vi "Multiple read.vi"(8 "error in (no error)":errorcluster, 9 "Data In":variant[](array[variant]), 10 "Section Names":string[](array[string]), 11 "Configuration File in":refnum<class "Configuration File.lvclass">) -> (0 "error out":errorcluster, 1 "Found section and keys?":bool[](array[boolean]), 2 "Data Out":variant[](array[variant]), 3 "Configuration File out":refnum<class "Configuration File.lvclass">)   [LabVIEW 2018, in "Configuration File.lvlib" / "Configuration File.lvclass"]
doc: "This VI reads multiple sections at once. Keeps the code clean."
uses:
  Configuration File.lvclass
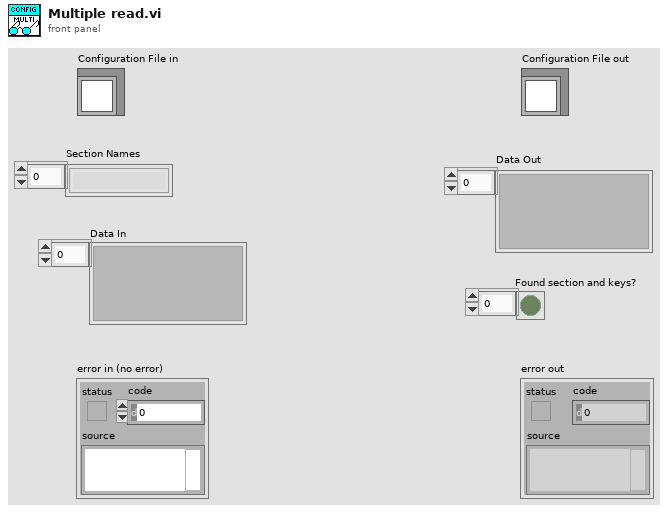
[diagram p1: front panel]
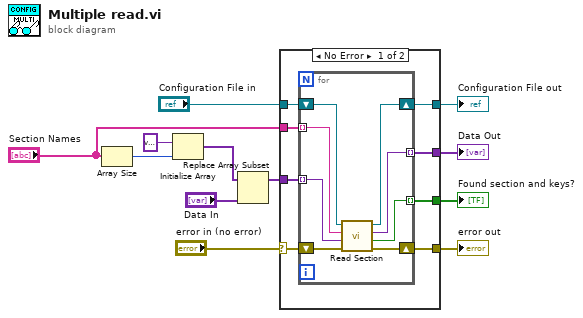
[diagram p0: block diagram]
diagram:
  n1 = Array Size(array="Section Names") -> (size(s)=w4:i32)
  n2 = Initialize Array(variant, w4) -> (w2:variant[])
  n3 = Replace Array Subset(array=w2, new element="Data In") -> (w3:variant[])  [unwired: 1 in]
  n4 = case shown="No Error" "error in (no error)" {
    selector: "error in (no error)" -> [w14 w31]
    tunnel: [w13 w31] -> w11
    tunnel: [w19 w30] -> w9
    tunnel: "Configuration File in" -> [w20 w30]
    tunnel: "Section Names" -> [w18 _]
    tunnel: w3 -> [w17 w29]
    tunnel: [w16 _] -> w8
    tunnel: [w15 w29] -> w7
    frame No Error {
      n5 = for {
        tunnel: w18 -> [w26] mode=indexing
        tunnel: w17 -> [w25] mode=indexing
        tunnel: [w24] -> w16 mode=indexing
        tunnel: [w23] -> w15 mode=indexing
        shift-right: [w27] -> w19
        shift-left: w20 -> [w28]
        shift-right: [w21] -> w13
        shift-left: w14 -> [w22]
        n6 = call-dynamic "Read Section.vi"("error in (no error)"=w22, "Data In"=w25, "Section Name"=w26, "Configuration File in"=w28) -> ("error out"=w21:errorcluster, "Found section and keys?"=w24:bool, "Data Out"=w23:variant, "Configuration File out"=w27:refnum<class "Configuration File.lvclass">)  [unwired: 4 in]
      }
    }
    frame Error {
    }
  }
  "error out" <- w11
  "Configuration File out" <- w9
  "Data Out" <- w7
  "Found section and keys?" <- w8
